vi "9211_Initialize.vi"(8 "error in (no error)":errorcluster, 9 "Slot Settings":T1, 11 "9211 in":refnum<class "9211.lvclass">) -> (0 "error out":errorcluster, 3 "9211 out":refnum<class "9211.lvclass">)   [LabVIEW 2011, in "Modules.lvlib" / "9211.lvclass"]
uses:
  9211.lvclass
  RSI Module/Slot Settings.ctl
  RSI Module/Module Models.ctl
  RSI Module/Channels.ctl
  RSI Module/Channel Type.ctl
  9211.lvclass/9211.ctl
  RSI Module/RSI Module.lvclass
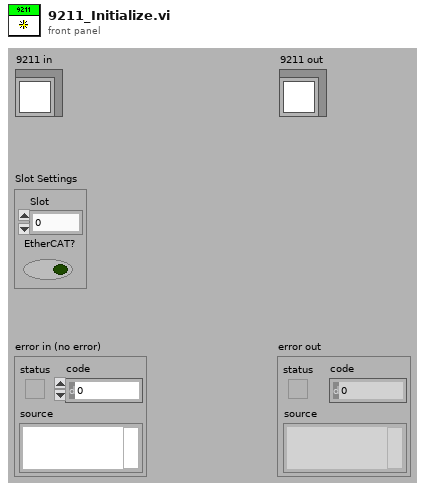
[diagram p1: front panel]
types:
  T1 = typedef "Modules.lvlib/RSI Module.lvclass/Slot Settings.ctl" = cluster{"Slot":u32, "EtherCAT?":bool}
  T2 = typedef "Modules.lvlib/RSI Module.lvclass/Module Models.ctl" = enum16{"Empty", "NI 9201", "NI 9203", "NI 9205", "NI 9206", "NI 9207", "NI 9208", "NI 9211", "NI 9213", "NI 9214", "NI 9215", "NI 9217", "NI 9219", "NI 9221", "NI 9225", "NI 9227", "NI 9229", "NI 9233", "NI 9234", "NI 9235", "NI 9236", "NI 9237", "NI 9239", "NI 9263", "NI 9264", "NI 9265", "NI 9269", "NI 9375", "NI 9401", "NI 9402", "NI 9403", "NI 9411", "NI 9421", "NI 9422", "NI 9423", "NI 9425", "NI 9426", "NI 9435", "NI 9472", "NI 9474", "NI 9475", "NI 9476", "NI 9477", "NI 9478", "NI 9481", "NI 9485"}
  T3 = typedef "Modules.lvlib/RSI Module.lvclass/Channels.ctl" = cluster{"# Input Channels":i32, "# Output Channels":i32, "Channel Type":T4, "Units":string}
  T4 = typedef "Modules.lvlib/RSI Module.lvclass/Channel Type.ctl" = enum16{"Analog", "Digital"}
  T5 = cluster{"Degree range":u32, "Thermocouple type":u32}
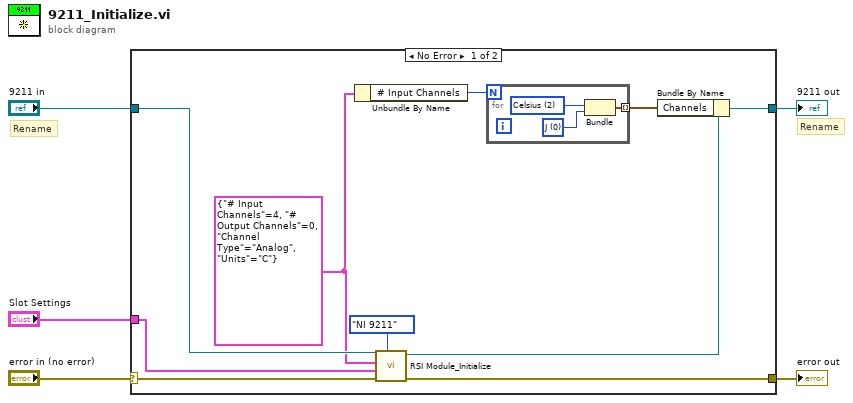
[diagram p0: block diagram]
diagram:
  # "Rename"
  # "Rename"
  n1 = case shown="No Error" "error in (no error)" {
    selector: "error in (no error)" -> [w13 w20]
    tunnel: [w12 w20] -> w4
    tunnel: [w10 w19] -> w2
    tunnel: "9211 in" -> [w15 w19]
    tunnel: "Slot Settings" -> [w14 _]
    frame No Error {
      w8 = T3 {"# Input Channels"=4, "# Output Channels"=0, "Channel Type"=enum."Analog", "Units"="C"} ("Channels")
      n2 = Unbundle By Name(w8) -> ("# Input Channels"=w7:i32)
      n3 = call "RSI Module_Initialize.vi"("Module Model"=Module_Models."NI 9211", "error in (no error)"=w13, "Slot Settings"=w14, "Channels"=w8, "RSI Module in"=w15) -> ("error out"=w12:errorcluster, "RSI Module out"=w11:refnum<class "9211.lvclass">)  [unwired: 5 in]
      n4 = for {
        N: w7 -> [_]
        tunnel: [w16] -> w6 mode=indexing
        w17 = u32 0 items=["J", "K", "T", "E", "R", "S", "N", "B"] ("Thermocouple type")
        w18 = u32 2 items=["Volts", "Kelvin", "Celsius", "Fahrenheit", "Rankine"] ("Degree range")
        n5 = Bundle("Degree range"=w18, "Thermocouple type"=w17) -> (w16:T5)  [unwired: 1 in]
      }
      n6 = Bundle By Name(cluster=w11, "Channels"=w6) -> (w10:refnum<class "9211.lvclass">)
    }
    frame Error {
    }
  }
  "error out" <- w4
  "9211 out" <- w2
